vi "MCL Cont Data Transactions List.vi"() -> (2 "Transactions":T1[](array[typedef]))   [LabVIEW 2013]
uses:
  Dataset Source.ctl
  Dataset Type.ctl
  Dataset Transaction Id.ctl
  Apps/Yes No Button.ctl
panel:
  in  "Dataset Types":T3[](array[typedef])=[enum."Displacement Command", enum."Displacement Command", enum."Displacement Command", enum."Displacement", enum."Displacement", enum."Displacement", enum."Force", enum."Force", enum."Force", enum."Actuator Command", enum."Actuator Command", enum."LVDT", enum."LVDT", enum."Load Cell", enum."Load Cell"]
  in  "Sources":T2[](array[typedef])=[enum."LBCB 1", enum."LBCB 2", enum."Combined", enum."LBCB 1", enum."LBCB 2", enum."Combined", enum."LBCB 1", enum."LBCB 2", enum."Combined", enum."LBCB 1", enum."LBCB 2", enum."LBCB 1", enum."LBCB 2", enum."LBCB 1", enum."LBCB 2"]
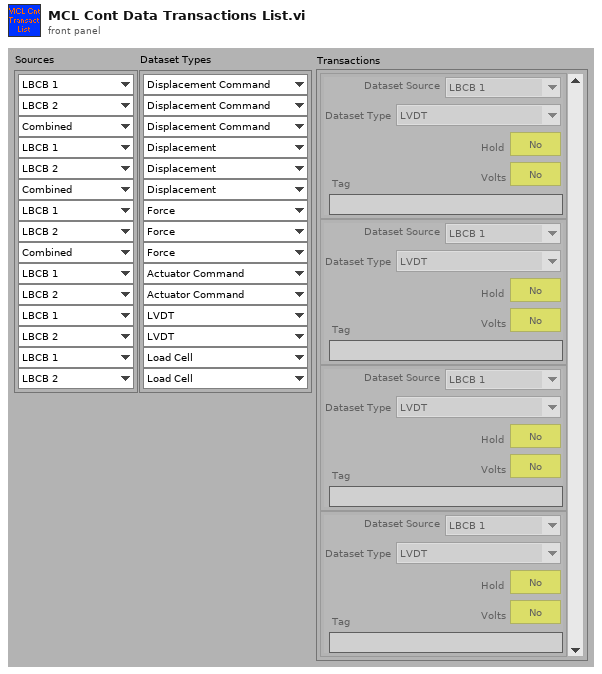
[diagram p1: front panel]
types:
  T1 = typedef "Dataset Transaction Id.ctl" = cluster{"Dataset Source":T2, "Dataset Type":T3, "Hold":T4, "Volts":T4, "Tag":string}
  T2 = typedef "Dataset Source.ctl" = enum16{"LBCB 1", "LBCB 2", "Combined", "External Sensors"}
  T3 = typedef "Dataset Type.ctl" = enum16{"LVDT", "Load Cell", "Actuator Command", "Servo Error", "Displacement Command", "Displacement", "Force"}
  T4 = typedef "Yes No Button.ctl" = bool
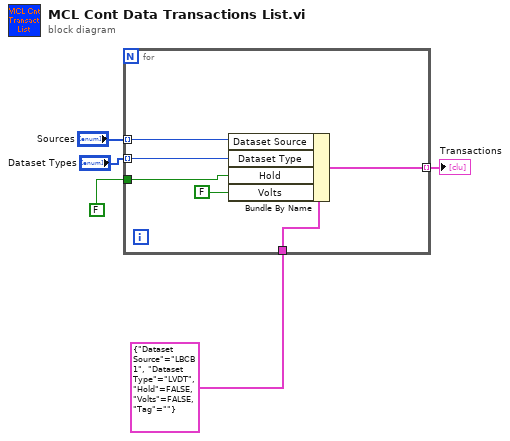
[diagram p0: block diagram]
diagram:
  n1 = for {
    tunnel: T1 {"Dataset Source"=enum."LBCB 1", "Dataset Type"=enum."LVDT", "Hold"=FALSE, "Volts"=FALSE, "Tag"=""} ("Dataset Trans Id") -> [w11]
    tunnel: "Sources" -> [w10] mode=indexing
    tunnel: "Dataset Types" -> [w9] mode=indexing
    tunnel: [w7] -> w2 mode=indexing
    tunnel: T4 FALSE ("Hold") -> [w6]
    n2 = Bundle By Name(cluster=w11, "Dataset Source"=w10, "Dataset Type"=w9, "Hold"=w6, "Volts"=T4 FALSE) -> (w7:T1)
  }
  "Transactions" <- w2
